vi "kvCanBusOn.vi"(2 "error in (no error)":errorcluster, 3 "Channel Handle (input only)":i32) -> (0 "error out":errorcluster, 1 "Channel Handle (ouput only)":i32)   [LabVIEW 2022 SP3]
doc: "Takes the specified circuit on-bus"
uses:
  canlib32.dll
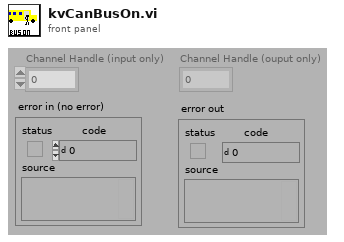
[diagram p1: front panel]
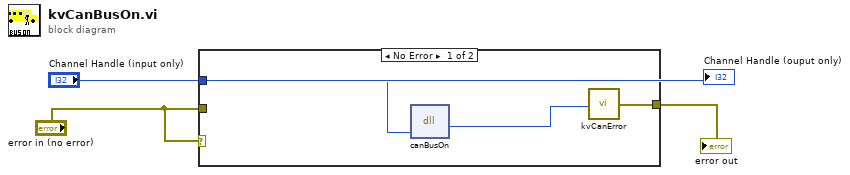
[diagram p0: block diagram]
diagram:
  n1 = case shown="No Error" "error in (no error)" {
    tunnel: [w6 w7] -> w3
    tunnel: "error in (no error)" -> [_ w7]
    tunnel: "Channel Handle (input only)" -> [w4 _]
    frame No Error {
      n2 = dll-call lib="canlib32.dll" fn="canBusOn" label="Call Library Function"("channelHandle"=w4) -> (w5:i32)  [unwired: 4 in, 2 out]
      n3 = call "kvCanError.vi"("error code"=w5) -> ("error out"=w6:errorcluster)
    }
    frame Error {
    }
  }
  "error out" <- w3
  "Channel Handle (ouput only)" <- "Channel Handle (input only)"
